vi "Stop and flush data stream.vi"(11 "FPGA Ref in":refnum<k20>) -> (3 "FPGA Ref out":refnum<k20>)   [LabVIEW 2018]
uses:
  <vilib>/rvi/interface/nirviMethod/nirviMethod.xnode
  FPGA/FPGA Main.vi
  <vilib>/rvi/errors/niLvFpgaMergeErrorWithErrorCode.vi
  FPGA Bitfiles/NewCompressorRig_FPGATarget_FPGAMain_d4D7mTAO5JM.lvbitx
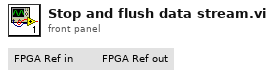
[diagram p1: front panel]
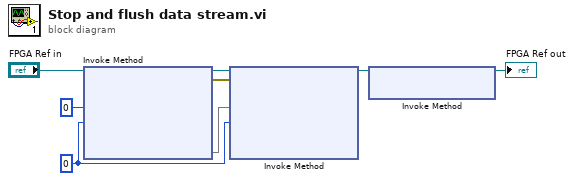
[diagram p0: block diagram]
diagram:
  w2 = 0 ("Timeout (ms)")
  n1 = xnode "Invoke Method"("FPGA VI Reference In"="FPGA Ref in", "Number of Elements"=u32 0, "Timeout (ms)"=w2) -> ("FPGA VI Reference Out"=w5:refnum<k20>, "error out"=w4:errorcluster, "Elements Remaining"=w3)  [unwired: 1 in, 1 out]
  n2 = xnode "Invoke Method"("FPGA VI Reference In"=w5, "error in"=w4, "Number of Elements"=w3, "Timeout (ms)"=w2) -> ("FPGA VI Reference Out"=w1:refnum<k20>)  [unwired: 3 out]
  n3 = xnode "Invoke Method"("FPGA VI Reference In"=w1) -> ("FPGA VI Reference Out"=→"FPGA Ref out":refnum<k20>)  [unwired: 1 in, 1 out]
